vi "Batch Enable Controls.vi"(7 "Mode":enum16{"Enable", "Disable"}(ring), 8 "error in (no error)":errorcluster, 11 "Control Refs":refnum<vi>[](array[refnum])) -> (0 "error out":errorcluster)   [LabVIEW 2015]
doc: "Enable or disable the entire group of controls specified."
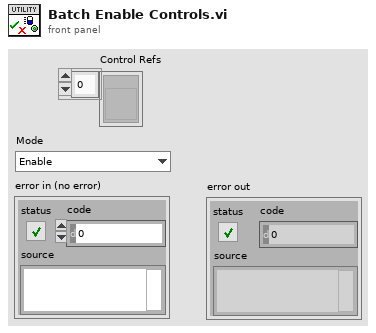
[diagram p1: front panel]
types:
  T1 = enum8{"Enabled", "Disabled", "Disabled and Grayed Out"}
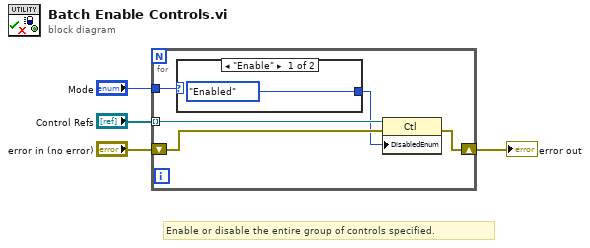
[diagram p0: block diagram]
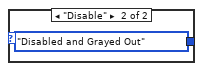
[diagram p2: hidden frame]
diagram:
  # "Enable or disable the entire group of controls specified."
  n1 = for {
    shift-right: [w8] -> w3
    shift-left: "error in (no error)" -> [w9]
    tunnel: "Control Refs" -> [w7] mode=indexing
    tunnel: "Mode" -> [w6]
    n2 = case shown="\"Enable\"" w6 {
      tunnel: [T1."Enabled" ("Disabled") T1."Disabled and Grayed Out" ("Disabled")] -> w5
      frame "Enable" {
      }
      frame "Disable" {
      }
    }
    n3 = property class="Ctl"(reference=w7, error in=w9, "DisabledEnum"=w5) -> (error out=w8:errorcluster)  [unwired: 1 out]
  }
  "error out" <- w3
